vi "Analog Read.vi"   [LabVIEW 2013, in "LVH-LINX.lvlib"]
doc: "Read the value of the specified analog input channel(s)."
uses:
  <vilib>/LabVIEW Hacker/LINX/LVH-LINX.lvlib
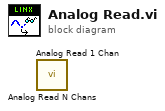
[diagram p0: block diagram]
diagram:
  n1 = call <vilib>:"Analog Read N Chans.vi"() -> ()  [unwired: 8 in, 4 out]
  n2 = call <vilib>:"Analog Read 1 Chan.vi"() -> ()  [unwired: 8 in, 4 out]
